vi "GEA2 Send Message.vi"(0 "GEA2 Reference In":refnum<k24>, 1 "Input Data":T1 {"Command" format="%02x"; "Destination" format="%02x"; "Source" format="%02x"}, 2 "# of Tries":u8=5 min=1, 5 "Timeout (ms)":u32=500, 7 "Wait for Acknowledgement?":bool, 11 "Error In":errorcluster) -> (4 "GEA2 Reference Out":refnum<k24>, 15 "Error Out":errorcluster)   [LabVIEW 2023, in "GEA2_Toolkit.lvlib"]
doc: "This VI sends a GEA2 message accross the GEA2 bus."
uses:
  library/GEA2_Toolkit.lvlib
  D:/Common/LabVIEW GEA2 Toolkit/source/GEA3 DLL Source/GeaCommunication.dll
  source/GEA3 DLL Source/GeaCommunication.dll
  type defs/Data In.ctl
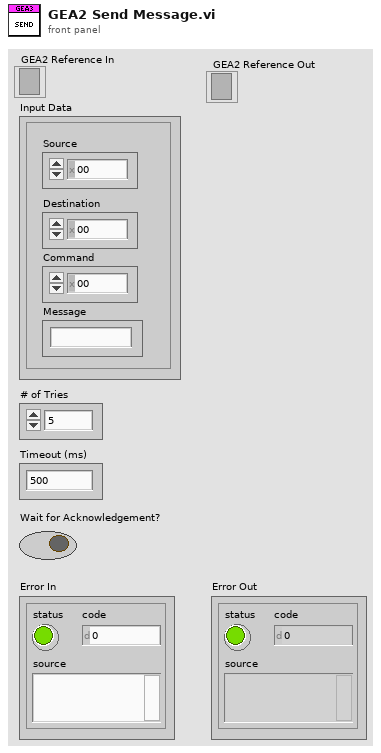
[diagram p1: front panel]
types:
  T1 = typedef "Data In.ctl" = cluster{"Source":u8, "Destination":u8, "Command":u8, "Message":string}
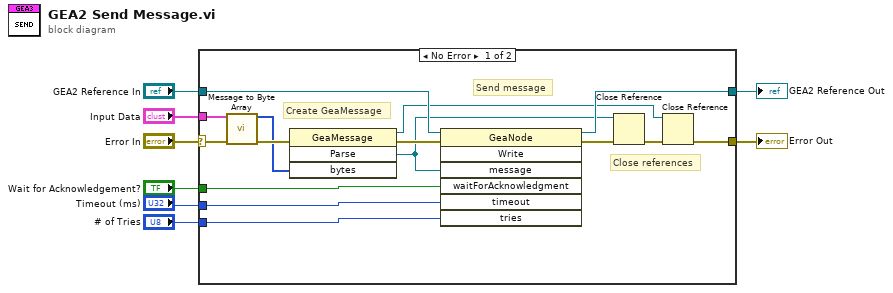
[diagram p0: block diagram]
diagram:
  n1 = case shown="No Error" "Error In" {
    selector: "Error In" -> [w17 w24]
    tunnel: "GEA2 Reference In" -> [w23 w25]
    tunnel: [w22 w25] -> w5
    tunnel: [w18 w24] -> w7
    tunnel: "# of Tries" -> [w12 _]
    tunnel: "Input Data" -> [w15 _]
    tunnel: "Timeout (ms)" -> [w13 _]
    tunnel: "Wait for Acknowledgement?" -> [w11 _]
    frame No Error {
      # "Close references"
      # "Send message"
      # "Create GeaMessage"
      n2 = call "Message to Byte Array.vi"("Input Data"=w15, "Error In"=w17) -> ("Byte Array"=w14:u8[], "Error Out"=w16:errorcluster)  [unwired: 12 in]
      n3 = invoke class="GeaMessage" method="Parse"(error in=w16, "bytes"=w14) -> (reference out=w9:refnum<k24>, error out=w20:errorcluster, "Parse"=w10:refnum<k24>)  [unwired: 2 in, 1 out]
      n4 = invoke class="GeaNode" method="Write"(reference=w23, error in=w20, "message"=w10, "waitForAcknowledgment"=w11, "timeout"=w13, "tries"=w12) -> (reference out=w22:refnum<k24>, error out=w21:errorcluster)  [unwired: 1 in, 5 out]
      n5 = Close Reference(reference=w10, error in (no error)=w21) -> (error out=w19:errorcluster)
      n6 = Close Reference(reference=w9, error in (no error)=w19) -> (error out=w18:errorcluster)
    }
    frame Error {
    }
  }
  "Error Out" <- w7
  "GEA2 Reference Out" <- w5
